vi "Parse Process Name.vi"(8 "error in (no error)":errorcluster, 10 "Process Name":string, 11 "Application In":refnum<class "Application.lvclass">) -> (0 "error out":errorcluster, 2 "Array":string[](array[string]), 3 "Application Out":refnum<class "Application.lvclass">)   [LabVIEW 2020, in "Application.lvclass"]
uses:
  Application.lvclass
  C:/Users/anton/Documents/GitHub/Triarc-Framework/source/Framework/Process/Process.lvclass
  Process/Process.lvclass
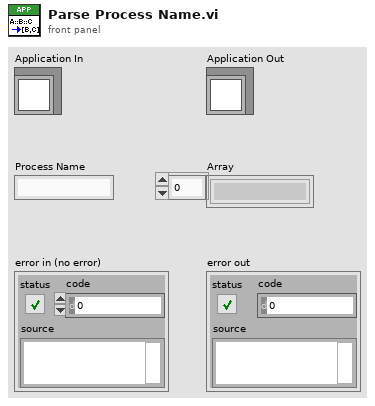
[diagram p1: front panel]
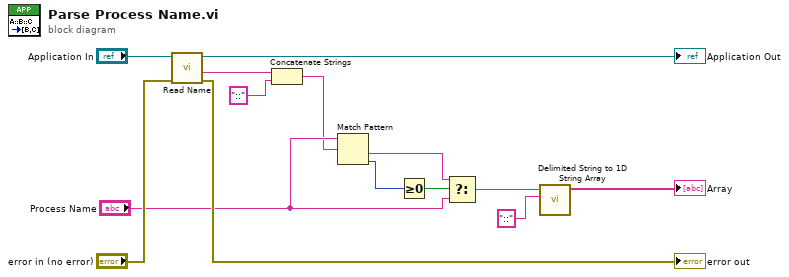
[diagram p0: block diagram]
diagram:
  n1 = call "Read Name.vi"("error in (no error)"="error in (no error)", "Process In"="Application In") -> ("error out"=→"error out":errorcluster, "Name"=w1:string, "Process Out"=→"Application Out":refnum<class "Application.lvclass">)  [unwired: 6 in, 1 out]
  n2 = Concatenate Strings(w1, "::" ("string")) -> (w6:string)
  n3 = Match Pattern(string="Process Name", regular expression=w6) -> (after substring=w7:string, offset past match=w10:i32)  [unwired: 1 in, 2 out]
  n4 = Greater Or Equal To 0?(x=w10) -> (x >= 0?=w9:bool)
  n5 = Select(t=w7, s=w9, f="Process Name") -> (s? t:f=w4:string)
  n6 = call <vilib>:"Delimited String to 1D String Array.vi"("delimiter"="::", "delimited string"=w4) -> ("string array"=→"Array":string[])  [unwired: 9 in]
